vi "Destroy.vi"(8 "error in (no error)":errorcluster, 11 "Barcode Detector in":refnum<class "Barcode Detector.lvclass">) -> (0 "error out":errorcluster)   [LabVIEW 2020, in "feature_detection.lvlib" / "Barcode Detector.lvclass"]
doc: "Destroy the Barcode Detector."
uses:
  Barcode Detector.lvclass
  Barcode Detector.lvclass/Barcode Detector.ctl
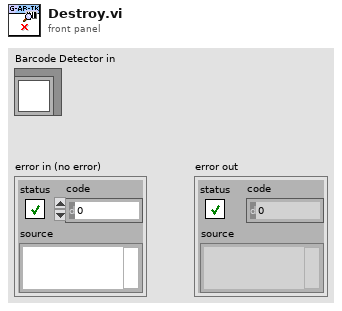
[diagram p1: front panel]
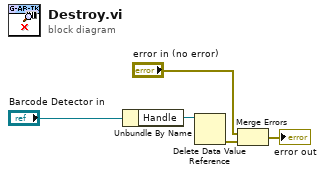
[diagram p0: block diagram]
diagram:
  n1 = Unbundle By Name("Barcode Detector in") -> ("Handle"=w5:refnum<data-value>)
  n2 = Delete Data Value Reference(data value reference=w5) -> (error out=w2:errorcluster)  [unwired: 1 in, 1 out]
  n3 = Merge Errors("error in (no error)", w2) -> (→"error out":errorcluster)
